vi "Pfeiffer Vacuum Turbo heat cool.vi"(8 "error in (no error)":errorcluster, 9 "PV Heating-Cooling - Cluster":T1={"Parameter"=0, "Parameter\nread only<->describe"=FALSE, "Pre-selection, heating\n  off     <-------->     on   "=TRUE, "TMS heating temperature\nset value [°C]"=40} {"TMS heating temperature\nset value [°C]" min=30 max=90 step=1; "Parameter" items=[" Pre-selection, heating [off / on]", " Heating TMS, actual value [°C] (read only)", " TMS regulator engaged [off/on] (read only)", " Maximum TMS temperature occured [°C] (read only)", " Heating type [conventional heating / TMS / cooling] (read only)", " TMS heating temperature set value [°C]"]}, 10 "Adress of unit":u16=1 min=1 max=999 step=1, 11 "COM Port Name in":refnum<visa-resource-name>="COM1") -> (0 "error out":errorcluster, 3 "response (data)":string)   [LabVIEW 2016]
doc: "This VI is an example of how to use the Pfeiffer Vacuum subVIs programmatically. This VI first initializes the instrument, takes measurements, then closes the instrument."
uses:
  Public/Turbopumps/PV Heating-Cooling - Cluster.ctl
  Pfeiffer Vacuum.lvlib
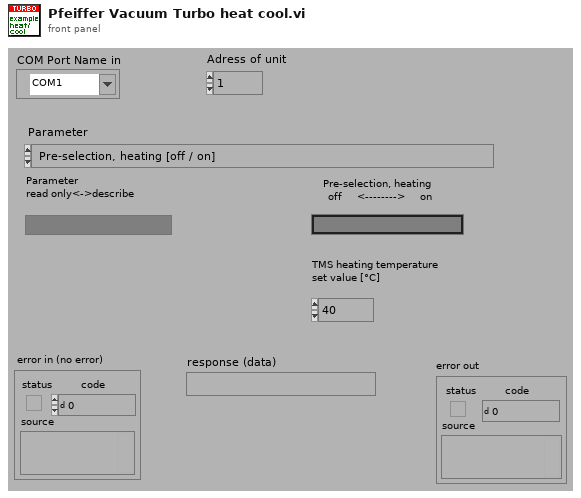
[diagram p1: front panel]
types:
  T1 = typedef "Pfeiffer Vacuum.lvlib/PV Heating-Cooling - Cluster.ctl" = cluster{"Parameter":u16, "Parameter\nread only<->describe":bool, "Pre-selection, heating\n  off     <-------->     on   ":bool, "TMS heating temperature\nset value [°C]":u16}
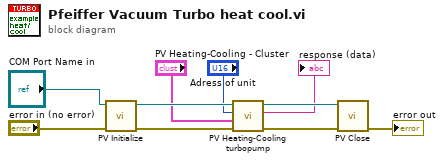
[diagram p0: block diagram]
diagram:
  n1 = call "PV Initialize.vi"("error in (no error)"="error in (no error)", "VISA session in"="COM Port Name in") -> ("error out"=w10:errorcluster, "VISA session out"=w8:refnum<visa-resource-name>)  [unwired: 8 in]
  n2 = call "PV Heating-Cooling turbopump.vi"("error in (no error)"=w10, "PV Heating-Cooling - Cluster"="PV Heating-Cooling - Cluster", "Adress of unit"="Adress of unit", "VISA session"=w8) -> ("error out"=w9:errorcluster, "response (data)"=→"response (data)":string, "dup VISA session"=w7:refnum<visa-resource-name>)  [unwired: 5 in]
  n3 = call "PV Close.vi"("VISA session"=w7, "error in (no error)"=w9) -> ("error out"=→"error out":errorcluster)  [unwired: 13 in]
